vi "allStatus.vi"(4 "intake":bool, 8 "gear":bool, 9 "shooter":bool, 10 "hopper1":bool, 11 "hopper0":bool) -> ()   [LabVIEW 2016]
uses:
  2ndContollerStatus.vi
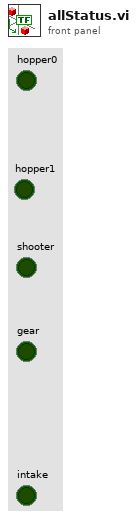
[diagram p1: front panel]
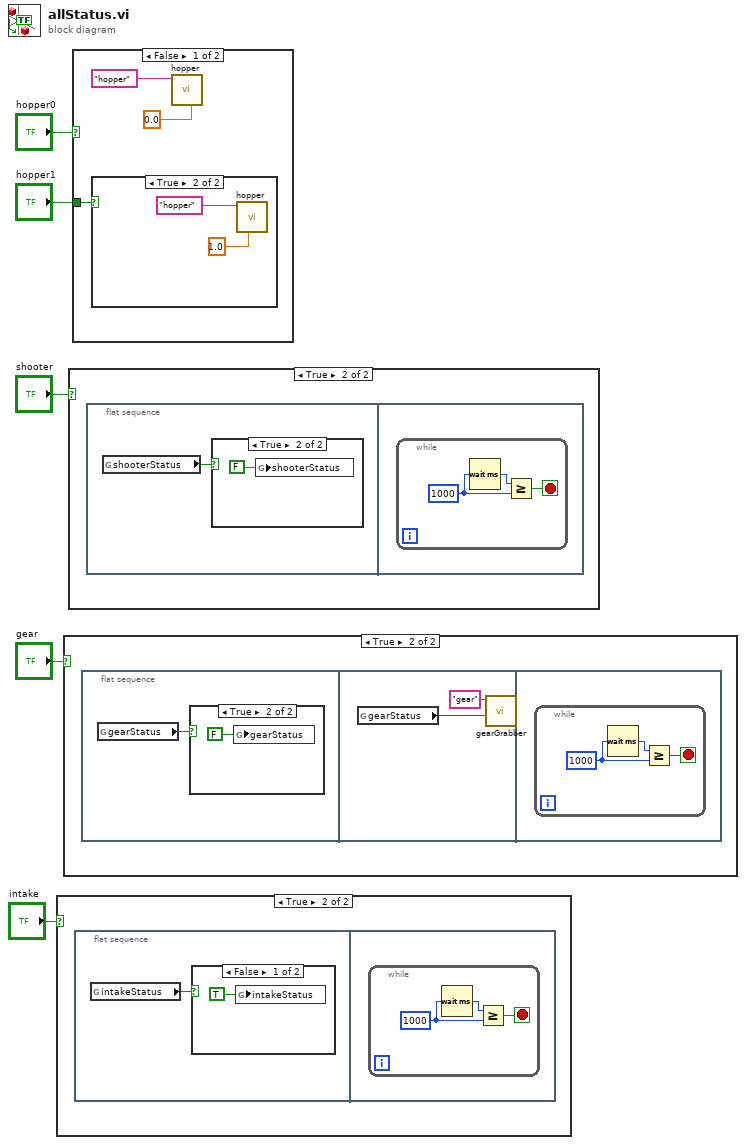
[diagram p0: block diagram]
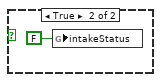
[diagram p3: hidden frame]
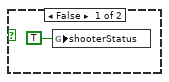
[diagram p5: hidden frame]
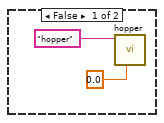
[diagram p6: hidden frame]
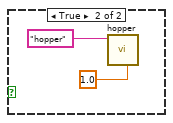
[diagram p7: hidden frame]
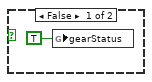
[diagram p9: hidden frame]
diagram:
  n1 = case shown="True" "intake" {
    frame False {
    }
    frame True {
      n2 = flat-sequence {
        frame #0 {
          n3 = global read "2ndContollerStatus.vi" "intakeStatus"() -> (w6:bool)
          n4 = case shown="False" w6 {
            frame False {
              n5 = global write "2ndContollerStatus.vi" "intakeStatus"(TRUE ("intakeStatus")) -> ()
            }
            frame True {
              n6 = global write "2ndContollerStatus.vi" "intakeStatus"(FALSE ("intakeStatus")) -> ()
            }
          }
        }
        frame #1 {
          n7 = while {
            stop <- w9 stop-if-true
            w11 = u32 1000 ("milliseconds to wait")
            n8 = Wait (ms)(milliseconds to wait=w11) -> (millisecond timer value=w10:u32)
            n9 = Greater Or Equal?(x=w10, y=w11) -> (x >= y?=w9:bool)
          }
        }
      }
    }
  }
  n10 = case shown="True" "gear" {
    frame False {
    }
    frame True {
      n11 = flat-sequence {
        frame #0 {
          n12 = global read "2ndContollerStatus.vi" "gearStatus"() -> (w12:bool)
          n13 = case shown="True" w12 {
            frame False {
              n14 = global write "2ndContollerStatus.vi" "gearStatus"(TRUE ("gearStatus")) -> ()
            }
            frame True {
              n15 = global write "2ndContollerStatus.vi" "gearStatus"(FALSE ("gearStatus")) -> ()
            }
          }
        }
        frame #1 {
          n16 = global read "2ndContollerStatus.vi" "gearStatus"() -> (w15:bool)
          n17 = call "gearGrabber.vi"("gearStatus"=w15, "gear"="gear") -> ()  [unwired: 9 in, 1 out]
        }
        frame #2 {
          n18 = while {
            stop <- w19 stop-if-true
            w17 = u32 1000 ("milliseconds to wait")
            n19 = Wait (ms)(milliseconds to wait=w17) -> (millisecond timer value=w18:u32)
            n20 = Greater Or Equal?(x=w18, y=w17) -> (x >= y?=w19:bool)
          }
        }
      }
    }
  }
  n21 = case shown="True" "shooter" {
    frame False {
    }
    frame True {
      n22 = flat-sequence {
        frame #0 {
          n23 = global read "2ndContollerStatus.vi" "shooterStatus"() -> (w20:bool)
          n24 = case shown="True" w20 {
            frame False {
              n25 = global write "2ndContollerStatus.vi" "shooterStatus"(TRUE ("shooterStatus")) -> ()
            }
            frame True {
              n26 = global write "2ndContollerStatus.vi" "shooterStatus"(FALSE ("shooterStatus")) -> ()
            }
          }
        }
        frame #1 {
          n27 = while {
            stop <- w23 stop-if-true
            w25 = u32 1000 ("milliseconds to wait")
            n28 = Wait (ms)(milliseconds to wait=w25) -> (millisecond timer value=w24:u32)
            n29 = Greater Or Equal?(x=w24, y=w25) -> (x >= y?=w23:bool)
          }
        }
      }
    }
  }
  n30 = case shown="False" "hopper0" {
    tunnel: "hopper1" -> [w28 _]
    frame False {
      n31 = case shown="True" w28 {
        frame False {
          n32 = call "hopper.vi"("Left axis value"=0.0 ("Right axis value"), "hopper"="hopper") -> ()  [unwired: 9 in, 1 out]
        }
        frame True {
          n33 = call "hopper.vi"("Left axis value"=1.0, "hopper"="hopper") -> ()  [unwired: 9 in, 1 out]
        }
      }
      n34 = call "hopper.vi"("Right axis value"=0.0, "hopper"="hopper") -> ()  [unwired: 9 in, 1 out]
    }
    frame True {
      n35 = call "hopper.vi"("Right axis value"=1.0, "hopper"="hopper") -> ()  [unwired: 9 in, 1 out]
    }
  }
